vi "Timer Clock Configuration.vi"(7 "Do Not Do Go()":bool, 8 "error in":errorcluster, 9 "Timer Clock Divisor":i32, 10 "Timer Clock Base":string, 11 "Handle In":i32) -> (0 "error out":errorcluster, 3 "Handle Out":i32)   [LabVIEW 2021]
panel:
  # "Timer Clock Base Strings:\n\nU3:\nLJ_tc2MHZ\nLJ_tc6MHZ\nLJ_tc24MHZ\nLJ_tc500KHZ_DIV\nLJ_tc2MHZ_DIV\nLJ_tc6MHZ_DIV\nLJ_tc24MHZ_DIV\n\nUE9:\nLJ_tc750KHZ\nLJ_tcSYS     //48MHz"
  # "(0-255 where 0=256)"
  # "If true, requests will be added but not executed.\nSince the UE9 does timer clock configuration\nand mode/value configuration in the same\nlow-level call, it could be useful in a time critical\napp to set this boolean true and put this VI\nbefore Timer Mode Configuration.vi, which will then\ndo the Go() that executes the requests from both VIs."
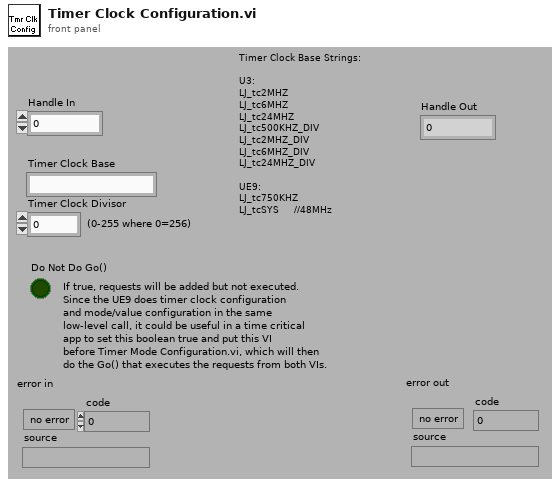
[diagram p1: front panel]
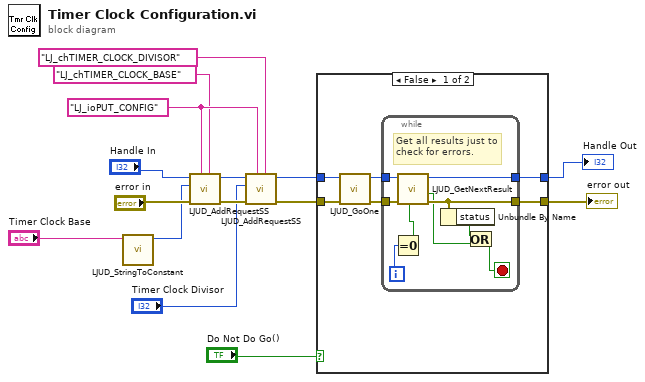
[diagram p0: block diagram]
diagram:
  w11 = "LJ_ioPUT_CONFIG" ("IOType")
  n1 = call "LJUD_StringToConstant.vi"("String"="Timer Clock Base") -> ("Constant Number"=w2:i32)  [unwired: 9 in, 1 out]
  n2 = call "LJUD_AddRequestSS.vi"("Channel"="LJ_chTIMER_CLOCK_BASE" ("IOType"), "IOType"=w11, "error in"="error in", "Value"=w2, "Handle In"="Handle In") -> ("error out"=w12:errorcluster, "Handle Out"=w13:i32)  [unwired: 5 in]
  n3 = call "LJUD_AddRequestSS.vi"("Channel"="LJ_chTIMER_CLOCK_DIVISOR" ("IOType"), "IOType"=w11, "error in"=w12, "Value"="Timer Clock Divisor", "Handle In"=w13) -> ("error out"=w6:errorcluster, "Handle Out"=w5:i32)  [unwired: 5 in]
  n4 = case shown="False" "Do Not Do Go()" {
    tunnel: [w19 w31] -> w15
    tunnel: [w18 w32] -> w14
    tunnel: w6 -> [w17 w31]
    tunnel: w5 -> [w16 w32]
    frame False {
      n5 = call "LJUD_GoOne.vi"("error in"=w17, "Handle In"=w16) -> ("error out"=w21:errorcluster, "Handle Out"=w20:i32)  [unwired: 8 in]
      n6 = while {
        tunnel: [w24] -> w18
        tunnel: [w26] -> w19
        tunnel: w20 -> [w27]
        tunnel: w21 -> [w28]
        i -> [w23]
        stop <- w30 stop-if-true
        # "Get all results just to\ncheck for errors."
        n7 = Equal To 0?(x=w23) -> (x = 0?=w29:bool)
        n8 = call "LJUD_GetNextResult.vi"("GetFirst"=w29, "error in"=w28, "Handle In"=w27) -> ("error out"=w26:errorcluster, "LJE_NO_MORE_DATA_AVAILABLE"=w22:bool, "Handle Out"=w24:i32)  [unwired: 3 in, 3 out]
        n9 = Unbundle By Name(w26) -> ("status"=w25:bool)
        n10 = Or(x=w25, y=w22) -> (x .or. y?=w30:bool)
      }
    }
    frame True {
    }
  }
  "error out" <- w15
  "Handle Out" <- w14
